vi "LoggerRef Get.vi"(8 "error in (no error)":errorcluster, 10 "LoggerRef Name":string) -> (0 "error out":errorcluster, 3 "LoggerRef Out":T1)   [LabVIEW 2014]
uses:
  LoggerRef.ctl
  <vilib>/Rock Robotics/WPI/Utilities/Refnum Registry Operation.ctl
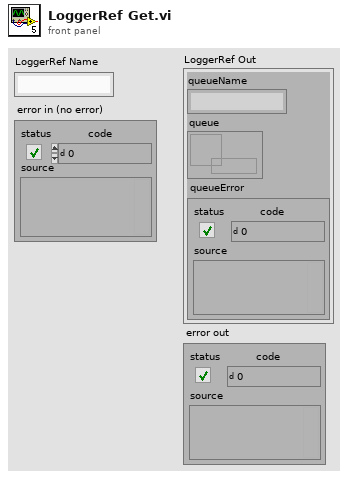
[diagram p1: front panel]
types:
  T1 = typedef "LoggerRef.ctl" = cluster{"queueName":string, "queue":refnum<queue>, "queueError":errorcluster}
  T2 = typedef "Refnum Registry Operation.ctl" = enum16{"set", "get", "delete", "get all names", "read name"}
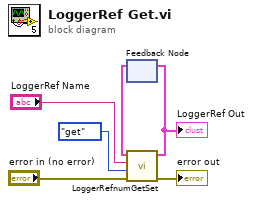
[diagram p0: block diagram]
diagram:
  n1 = feedback #1() -> (w1:T1)  [unwired: 1 in]
  n2 = call "LoggerRefnumGetSet.vi"("Logger Error In (no error)"="error in (no error)", "menu"=Refnum_Registry_Operation."get", "Logger Ref Name"="LoggerRef Name", "LoggerRef In"=w1) -> ("Logger Error Out"=→"error out":errorcluster, "LoggerRef 2 Out"=w2:T1)  [unwired: 5 in, 1 out]
  "LoggerRef Out" <- w2
  n3 = feedback-in #1(w2) -> ()
